vi "Metrolab_main_SF_and_dipoles_THM1176.vi"() -> ()   [LabVIEW 2020]
uses:
  <vilib>/Analysis/baseanly.llb/Mean (DBL).vi
  <vilib>/Analysis/NI_AALBase.lvlib
panel:
  out "Error out":errorcluster
  out "Output":T1={"X"=[-0.192], "Y"=[-0.056], "Z"=[0.117], "Temperature"=0, "Timestamp"=525.141756172, "Digits"=3} {"Z" format="%.5f"; "Y" format="%.5f"; "X" format="%.5f"}
  in  "Select":T2={"X"=TRUE, "Y"=TRUE, "Z"=TRUE, "Temp"=FALSE, "Timstamp"=FALSE}
  in  "VISA resource":refnum<visa-resource-name>="USB0::0x1BFA::0x0498::0002759::INSTR"
  out "XY Graph 2":cluster{dbl[], dbl[]}(graph)
  out "Labels":string[](array[string])=["I_D1 (A)", "I_D2(A)", "I_SFDC (A)", "I_RF (A)", "l (mm)", "z (mm)", "Bx (mT)", "By (mT)", "Bz (mT)", "|B| (mT)"]
  in  "I_D2 (A)":dbl=112.0
  in  "I_D1 (A)":dbl
  out "Graph (Bx)":cluster{timestamp[], dbl[]}(graph)={[timestamp(3793092767.9882584 s since 1904-01-01), timestamp(3793092775.7172394 s since 1904-01-01)], [-0.191, -0.192]} caption="XY Graph"
  out "XY Graph":cluster{dbl[], dbl[]}(graph)={[112.0, 112.0], [590.0, 580.0]}
  in  "I_RF (A)":dbl
  in  "I_SFDC (A)":dbl=112.0
  out "Cycle #":i32=1
  in  "COMMENT":string="BDC_z_reverse_D1_0A_D2_0A_SFDC_3A5"
  out "Graph (Bz)":cluster{timestamp[], dbl[]}(graph)={[timestamp(3793092767.9882584 s since 1904-01-01), timestamp(3793092775.7172394 s since 1904-01-01)], [0.121, 0.117]} caption="XY Graph"
  out "Graph (By)":cluster{timestamp[], dbl[]}(graph)={[timestamp(3793092767.9882584 s since 1904-01-01), timestamp(3793092775.7172394 s since 1904-01-01)], [-0.056, -0.056]} caption="XY Graph"
  in  "Stop":bool
  out "Graph (z)":cluster{timestamp[], dbl[]}(graph)={[timestamp(3793092767.9882584 s since 1904-01-01), timestamp(3793092775.7172394 s since 1904-01-01)], [590.0, 580.0]} caption="XY Graph"
  out "Z (mm) = 600 - L":dbl=580.0 format="%_5f"
  in  "L (mm)":dbl=20.0
  in  "Measure":bool
  out "File Error Out":errorcluster
  in  "base path":path=path "C:/LabVIEW/DATA/J-PARC_202403"
  out "error out":errorcluster caption="エラー出力" {"code" format="%.0x"}
  out "Results":dbl[](array[numeric])=[112.0, 112.0, 112.0, 0.0, 20.0, 580.0, -0.192, -0.056, 0.117, 0.23170886905770352] format="%_4f"
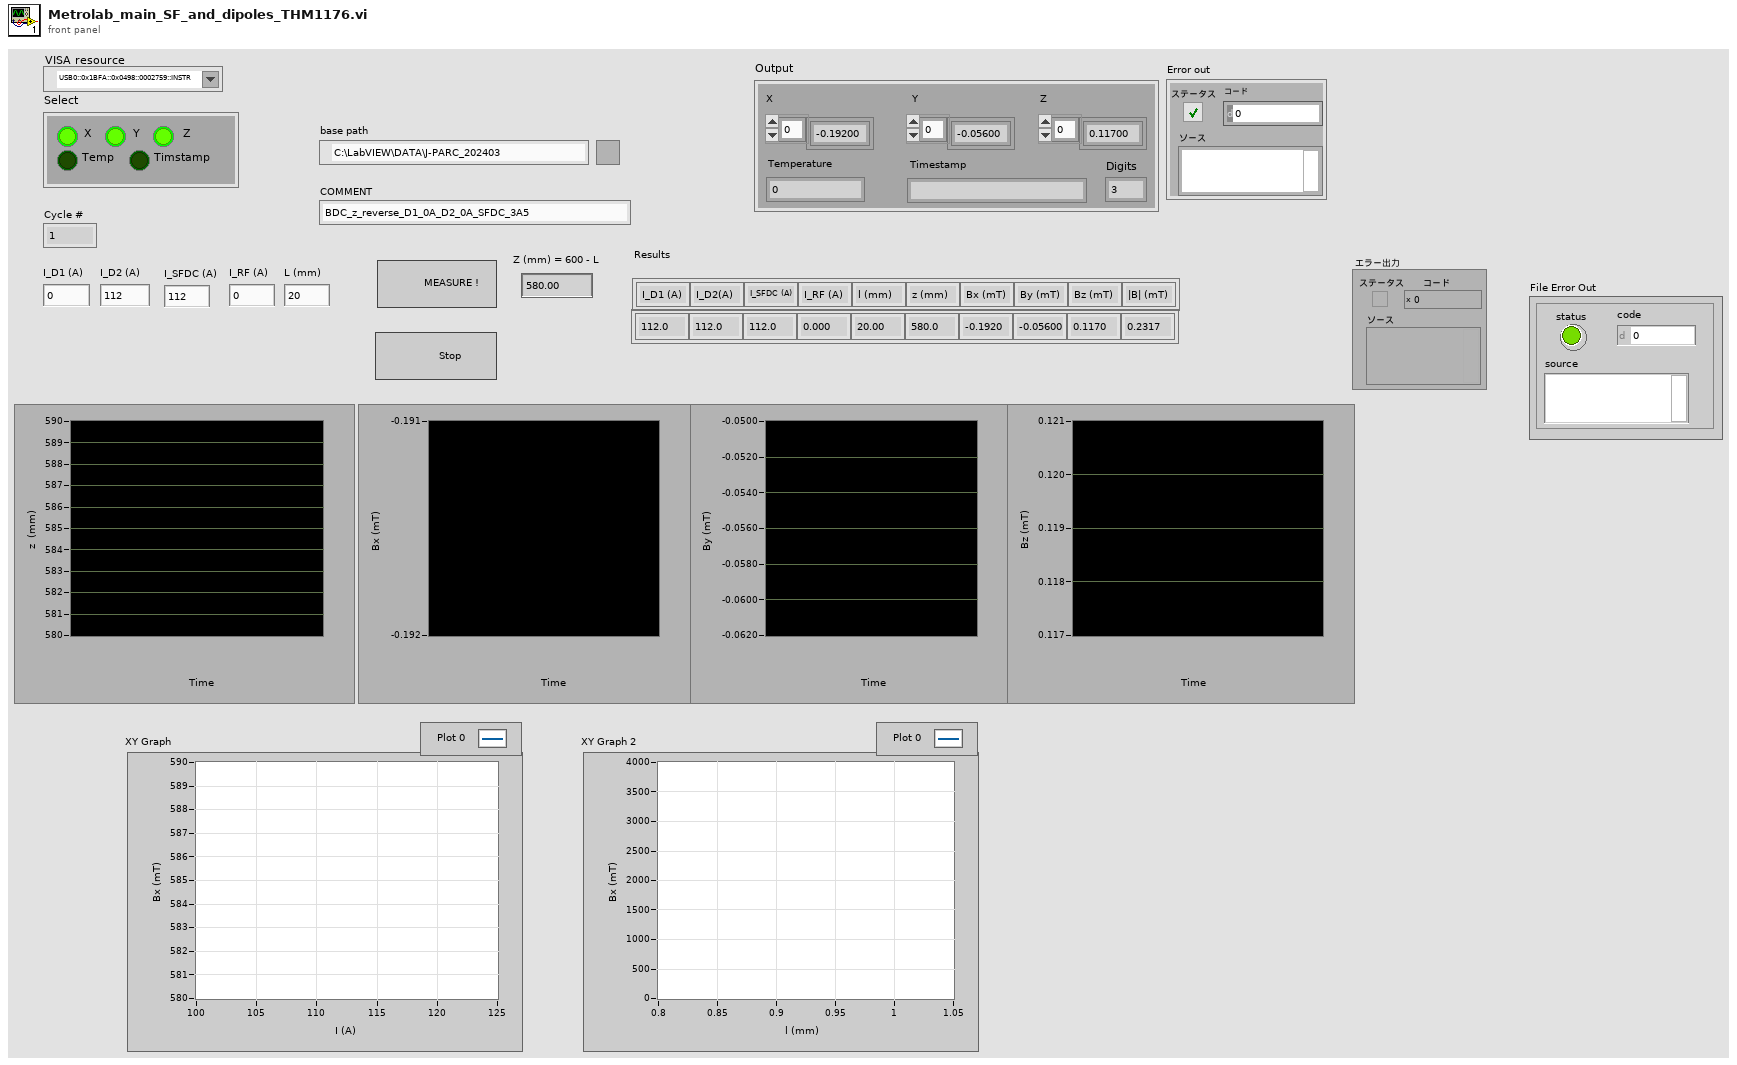
[diagram p1: front panel]
types:
  T1 = cluster{"X":dbl[], "Y":dbl[], "Z":dbl[], "Temperature":u16, "Timestamp":ext, "Digits":u8}
  T2 = cluster{"X":bool, "Y":bool, "Z":bool, "Temp":bool, "Timstamp":bool}
  T3 = enum16{"open", "replace", "create", "open or create", "replace or create", "replace or create with confirmation"}
  T4 = enum16{"Setup", "Setup query", "INITiate", "ABORt"}
  T5 = enum16{"Set units", "Units query", "Units all query"}
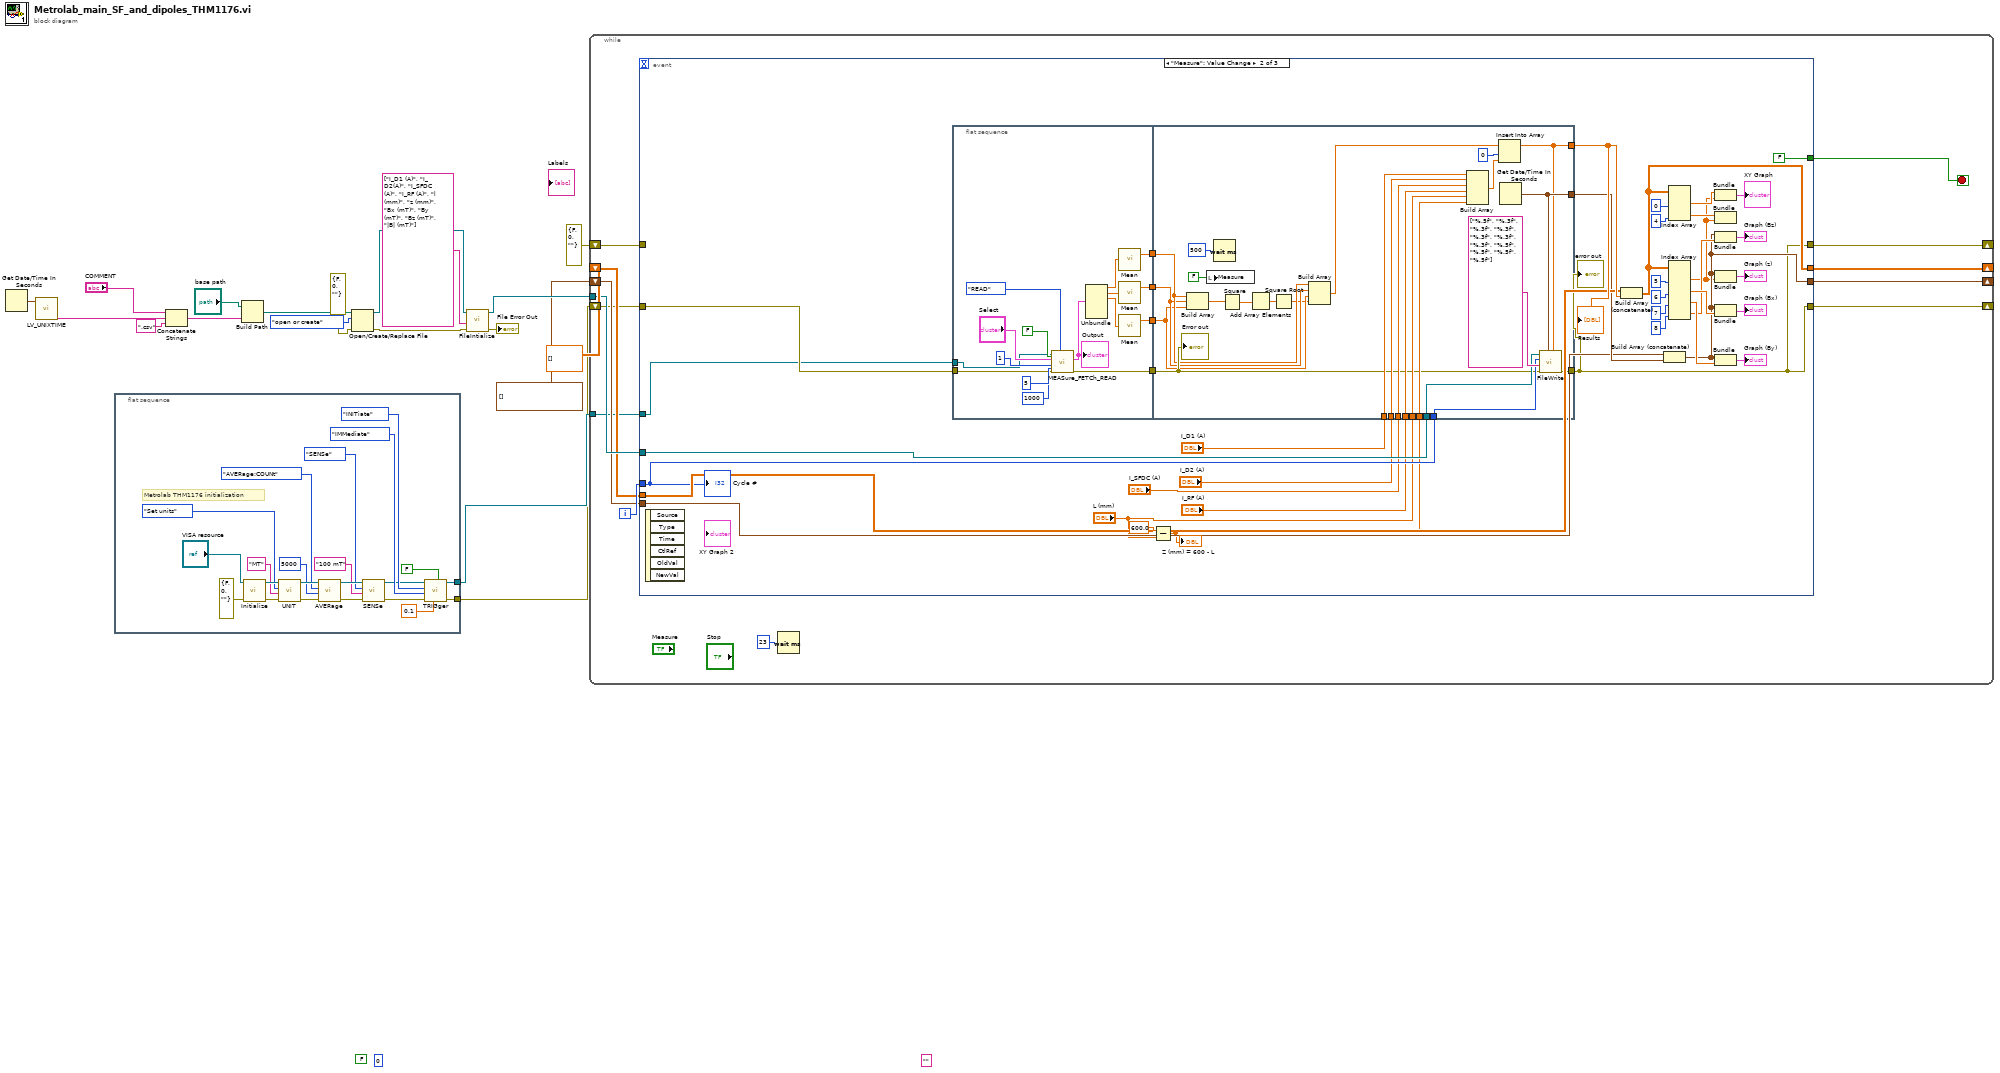
[diagram p0: block diagram]
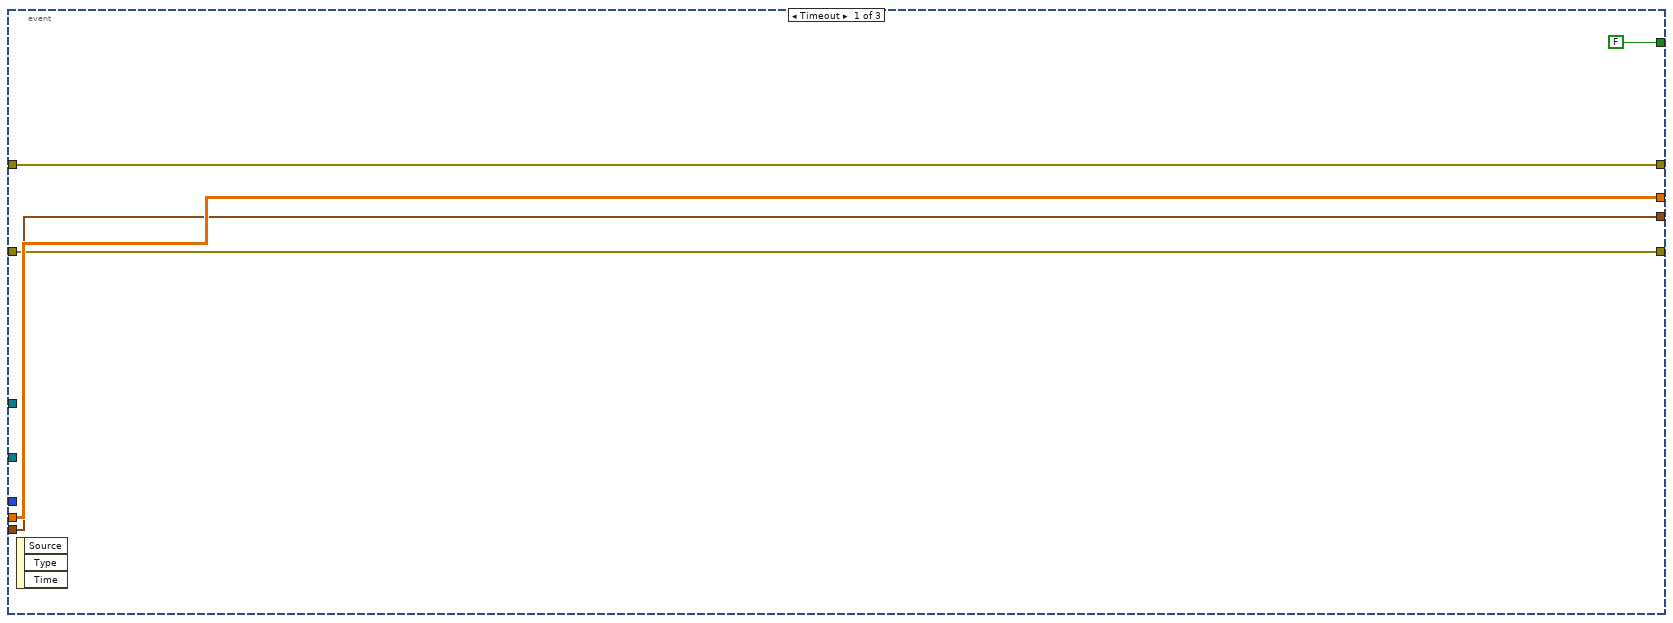
[diagram p2: hidden frame]
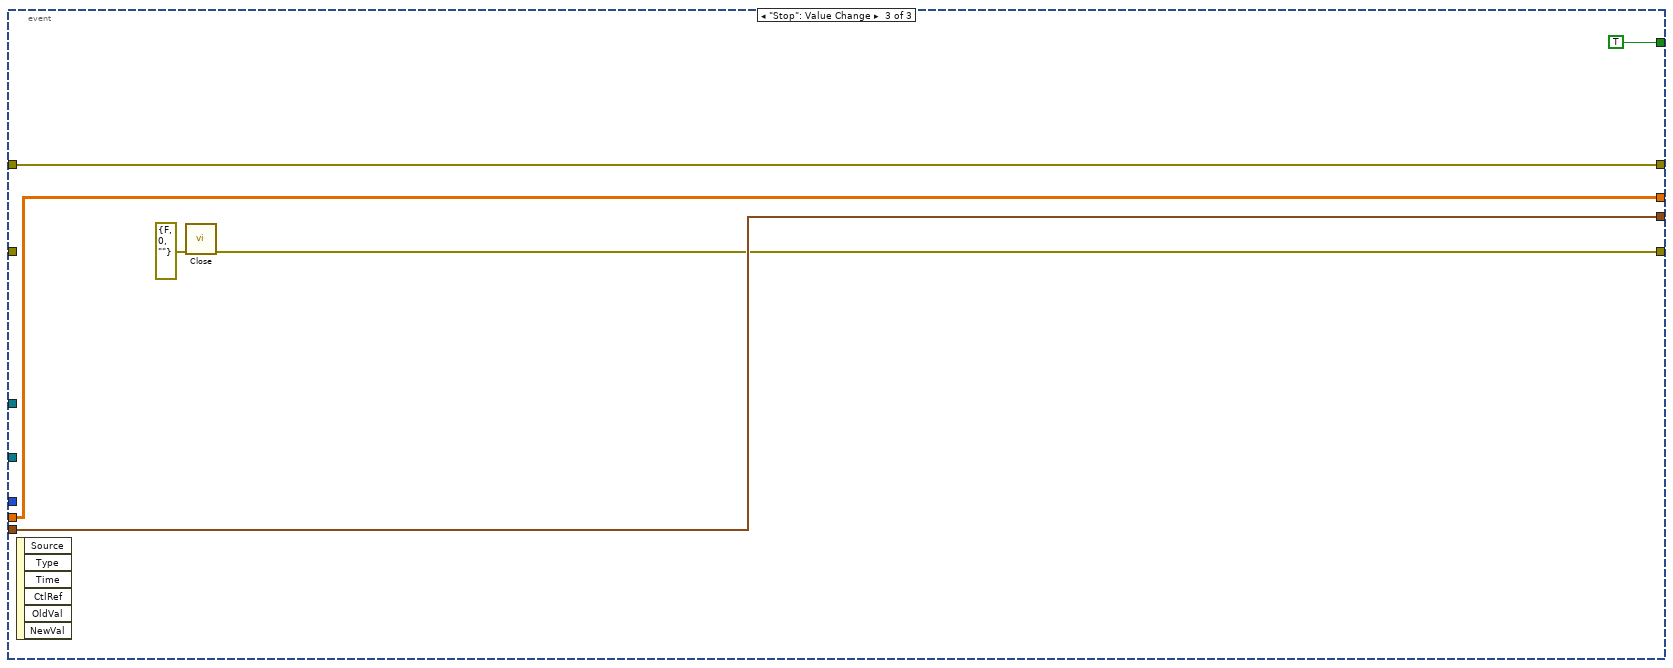
[diagram p3: hidden frame]
diagram:
  (unwired) FALSE ("status")
  (unwired) 0 ("code")
  (unwired) "" ("source")
  n1 = Get Date/Time In Seconds() -> (seconds since 1Jan1904=w17:timestamp)
  n2 = call "LV_UNIXTIME.vi"("current time"=w17) -> ("date/time string"=w14:string)  [unwired: 9 in, 1 out]
  n3 = flat-sequence {
    tunnel: [w27] -> w2
    tunnel: [w26] -> w1
    frame #0 {
      # "Metrolab THM1176 initialization"
      n4 = call "Initialize.vi"("Error in (no error)"=errorcluster {"status"=FALSE, "code"=0, "source"=""}, "VISA resource"="VISA resource") -> ("Error out"=w38:errorcluster, "Dup VISA resource"=w39:refnum<visa-resource-name>)  [unwired: 3 in, 5 out]
      n5 = call "UNIT.vi"("Error in (no error)"=w38, "Units"="MT", "Function"=T5."Set units", "VISA resource"=w39) -> ("Error out"=w34:errorcluster, "Dup VISA resource"=w35:refnum<visa-resource-name>)  [unwired: 5 in, 1 out]
      n6 = call "AVERage.vi"("Error in (no error)"=w34, "Count"=u16 5000, "Function"=enum16{"AVERage:COUNt query", "AVERage:COUNt"}."AVERage:COUNt", "VISA resource"=w35) -> ("Error out"=w25:errorcluster, "Dup VISA resource"=w22:refnum<visa-resource-name>)  [unwired: 5 in, 1 out]
      n7 = call "SENSe.vi"("Error in (no error)"=w25, "Range"="100 mT", "Function"=enum16{"SENSe", "SENSe Query"}."SENSe", "VISA resource"=w22) -> ("Error out"=w24:errorcluster, "Dup VISA resource"=w23:refnum<visa-resource-name>)  [unwired: 4 in, 2 out]
      n8 = call "TRIGger.vi"("Continuous"=FALSE, "Period (s)"=0.1, "Error in (no error)"=w24, "Source"=enum16{"IMMediate", "TIMer", "BUS"}."IMMediate", "Function"=T4."INITiate", "VISA resource"=w23) -> ("Error out"=w26:errorcluster, "Dup VISA resource"=w27:refnum<visa-resource-name>)  [unwired: 3 in, 1 out]
    }
  }
  n9 = Concatenate Strings("COMMENT", w14, ".csv" ("string")) -> (w12:string)
  n10 = Build Path(base path="base path", name or relative path=w12) -> (appended path=w16:path)
  n11 = Open/Create/Replace File(file path (use dialog)=w16, error in=errorcluster {"status"=FALSE, "code"=0, "source"=""} ("エラー入力"), operation (0:open)=T3."open or create") -> (refnum out=w9:refnum<file>, error out=w10:errorcluster)  [unwired: 3 in, 1 out]
  n12 = call "FileIntialize.vi"("Error In"=w10, "Labels"=string[] ["I_D1 (A)", "I_D2(A)", "I_SFDC (A)", "I_RF (A)", "l (mm)", "z (mm)", "Bx (mT)", "By (mT)", "Bz (mT)", "|B| (mT)"], "refnum in"=w9) -> ("Error Out"=→"File Error Out":errorcluster, "File Refnum"=w7:refnum<file>)  [unwired: 7 in]
  n13 = while {
    tunnel: w7 -> [w53]
    shift-right: [w51] -> _
    shift-left: errorcluster {"status"=FALSE, "code"=0, "source"=""} ("Error Out") -> [w50]
    shift-right: [w48] -> _
    shift-left: dbl[][] [] -> [w49]
    shift-right: [w47] -> _
    shift-left: timestamp[] [] -> [w46]
    shift-right: [w43] -> _
    shift-left: w1 -> [w44]
    tunnel: w2 -> [w42]
    i -> [w52]
    stop <- w45 stop-if-true
    n14 = event shown="[1] \"Measure\": Value Change" {
      selector: _ -> [_ _ _]
      dyn-events: _ -> [_ _ _]
      timeout: _ -> [_ _ _]
      tunnel: w53 -> [_ w92 _]
      tunnel: w52 -> [_ w91 _]
      tunnel: [w59 w64 w143] -> w51
      tunnel: w50 -> [w59 _ w143]
      tunnel: w49 -> [w58 w97 w145]
      tunnel: [w58 w81 w145] -> w48
      tunnel: [w56 w73 w144] -> w47
      tunnel: w46 -> [w56 w90 w144]
      tunnel: [FALSE ("Stop") FALSE ("Stop") TRUE ("Stop")] -> w45
      tunnel: w44 -> [w55 w66 _]
      tunnel: [w55 w64 w142] -> w43
      tunnel: w42 -> [_ w60 _]
      event Timeout {
        n15 = event-data() -> ()  [unwired: 1 in, 3 out]
      }
      event "Measure": Value Change {
        n16 = event-data() -> ()  [unwired: 1 in, 6 out]
        n17 = flat-sequence {
          tunnel: w66 -> [w100]
          tunnel: [w110] -> w65
          tunnel: [w106] -> w63
          tunnel: [w104] -> w62
          tunnel: [w102] -> w61
          tunnel: w60 -> [w101]
          tunnel: [w128] -> w98
          tunnel: [w139] -> w64
          tunnel: [w138] -> w93
          tunnel: w92 -> [w137]
          tunnel: w91 -> [w136]
          tunnel: "L (mm)" -> [w135]
          tunnel: w87 -> [w134]
          tunnel: "I_SFDC (A)" -> [w131]
          tunnel: "I_RF (A)" -> [w130]
          tunnel: "I_D1 (A)" -> [w127]
          tunnel: "I_D2 (A)" -> [w126]
          tunnel: w65 -> [w124]
          tunnel: w63 -> [w120]
          tunnel: w62 -> [w119]
          tunnel: w61 -> [w118]
          frame #0 {
            n18 = call "MEASure_FETCh_READ.vi"("Timeout (ms)"=u32 1000, "Sleep"=FALSE, "Digits"=u8 5, "Function"=enum16{"MEASure", "READ", "FETCh"}."READ", "Error in (no error)"=w100, "Size"=u16 1, "Select"="Select", "VISA resource"=w101) -> ("Error out"=w110:errorcluster, "Output"=w108:T1)  [unwired: 1 in, 1 out]
            "Output" <- w108
            n19 = Unbundle(w108) -> ("X"=w107:dbl[], "Y"=w105:dbl[], "Z"=w103:dbl[])  [unwired: 3 out]
            n20 = call-poly <vilib>:"Mean.vi"("X"=w107) -> ("mean"=w106:dbl)  [unwired: 1 out]
            n21 = call-poly <vilib>:"Mean.vi"("X"=w105) -> ("mean"=w104:dbl)  [unwired: 1 out]
            n22 = call-poly <vilib>:"Mean.vi"("X"=w103) -> ("mean"=w102:dbl)  [unwired: 1 out]
          }
          frame #1 {
            n23 = Build Array(w120, w119, w118) -> (w123:dbl[])
            n24 = local write "Measure"(FALSE ("Value (Signaling)")) -> ()
            n25 = Wait (ms)(milliseconds to wait=u32 500 ("ミリ秒待機時間")) -> ()  [unwired: 1 out]
            n26 = Square(x=w123) -> (x^2=w122:dbl[])
            n27 = Add Array Elements(numeric array=w122) -> (sum=w121:dbl)
            n28 = Square Root(x=w121) -> (sqrt(x)=w117:dbl)
            n29 = Build Array(w120, w119, w118, w117) -> (w125:dbl[])
            n30 = Build Array(w127, w126, w131, w130, w135, w134) -> (w129:dbl[])
            n31 = Insert Into Array(array=w125, index=0, new element=w129) -> (w128:dbl[])
            n32 = Get Date/Time In Seconds() -> (seconds since 1Jan1904=w138:timestamp)
            n33 = call "FileWrite.vi"("DataArray"=w128, "Time Stamp"=w138, "Error In"=w124, "FileFormat"=string[] ["%.5f", "%.3f", "%.3f", "%.3f", "%.3f", "%.3f", "%.3f", "%.5f", "%.5f", "%.5f", "%.5f"], "Index"=w136, "refnum in"=w137) -> ("Error Out"=w139:errorcluster)  [unwired: 4 in, 1 out]
            "Error out" <- w124
          }
        }
        n34 = Subtract(x=600.0, y="L (mm)") -> (x-y=w87:dbl)
        "Z (mm) = 600 - L" <- w87
        n35 = Build Array (concatenate)(w97, w98) -> (w81:dbl[][])
        n36 = Build Array (concatenate)(w90, w93) -> (w73:timestamp[])
        n37 = Index Array(array=w81, index (col) #1=0 ("disabled index (col)"), index (col) #2=4 ("指標 （列）")) -> (element #1=w69:dbl[], element #2=w68:dbl[])  [unwired: 2 in]
        n38 = Index Array(array=w81, index (col) #1=5 ("disabled index (col)"), index (col) #2=6 ("disabled index (col)"), index (col) #3=7 ("disabled index (col)"), index (col) #4=8 ("index (col)")) -> (element #1=w67:dbl[], element #2=w85:dbl[], element #3=w84:dbl[], element #4=w77:dbl[])  [unwired: 4 in]
        n39 = Bundle(w69, w67) -> (→"XY Graph":cluster{dbl[], dbl[]})  [unwired: 1 in]
        n40 = Bundle(w68, w67) -> ()  [unwired: 1 in, 1 out]
        n41 = Bundle(w73, w77) -> (→"Graph (Bz)":cluster{timestamp[], dbl[]})  [unwired: 1 in]
        n42 = Bundle(w73, w67) -> (→"Graph (z)":cluster{timestamp[], dbl[]})  [unwired: 1 in]
        n43 = Bundle(w73, w85) -> (→"Graph (Bx)":cluster{timestamp[], dbl[]})  [unwired: 1 in]
        n44 = Bundle(w73, w84) -> (→"Graph (By)":cluster{timestamp[], dbl[]})  [unwired: 1 in]
        "Results" <- w98
        "error out" <- w64
        "Cycle #" <- w91
      }
      event "Stop": Value Change {
        n45 = event-data() -> ()  [unwired: 1 in, 6 out]
        n46 = call "Close.vi"("Error in (no error)"=errorcluster {"status"=FALSE, "code"=0, "source"=""}) -> ("Error out"=w142:errorcluster)  [unwired: 10 in]
      }
    }
    n47 = Wait (ms)(milliseconds to wait=u32 23) -> ()  [unwired: 1 out]
  }
